vi "SetIncrementTime.vi"(8 "error in":errorcluster, 11 "Cycles":T1={"DELICATE"=10.0, "LOW"=10.0, "MEDIUM"=10.0, "HIGH"=10.0} {"HIGH" min=0.0 max=90.0 step=1.0; "MEDIUM" min=0.0 max=90.0 step=1.0; "LOW" min=0.0 max=90.0 step=1.0; "DELICATE" min=0.0 max=90.0 step=1.0}) -> (0 "error out":errorcluster, 3 "TimeData":string)   [LabVIEW 2023]
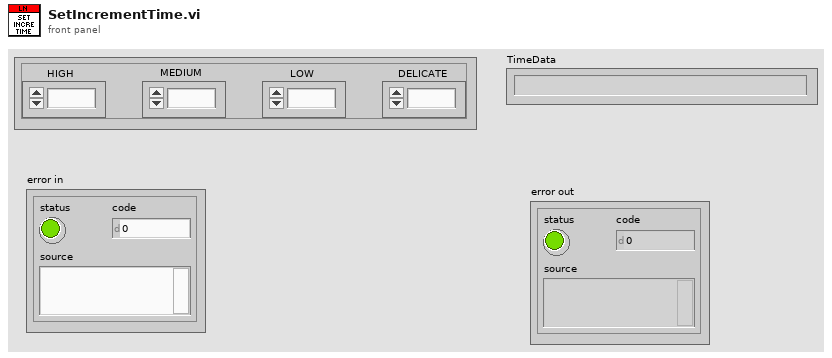
[diagram p1: front panel]
types:
  T1 = cluster{"DELICATE":dbl, "LOW":dbl, "MEDIUM":dbl, "HIGH":dbl}
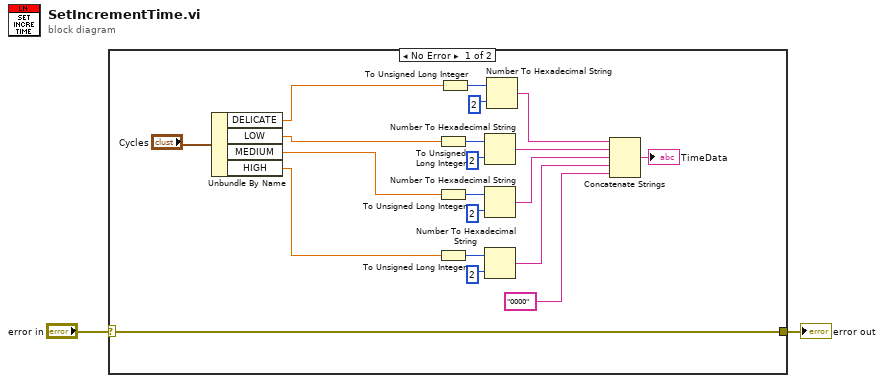
[diagram p0: block diagram]
diagram:
  n1 = case shown="No Error" "error in" {
    selector: "error in" -> [w3 w23]
    tunnel: [w3 w23] -> w1
    frame No Error {
      n2 = Unbundle By Name("Cycles") -> ("DELICATE"=w7:dbl, "LOW"=w6:dbl, "MEDIUM"=w5:dbl, "HIGH"=w4:dbl)
      n3 = To Unsigned Long Integer(number=w6) -> (unsigned 32bit integer=w20:u32)
      n4 = To Unsigned Long Integer(number=w5) -> (unsigned 32bit integer=w17:u32)
      n5 = To Unsigned Long Integer(number=w4) -> (unsigned 32bit integer=w16:u32)
      n6 = To Unsigned Long Integer(number=w7) -> (unsigned 32bit integer=w21:u32)
      n7 = Number To Hexadecimal String(1:i16 2 ("width (-)"), 2:w20) -> (0:w13:string)
      n8 = Number To Hexadecimal String(1:i16 2 ("width (-)"), 2:w17) -> (0:w12:string)
      n9 = Number To Hexadecimal String(1:i16 2 ("width (-)"), 2:w16) -> (0:w11:string)
      n10 = Number To Hexadecimal String(1:i16 2 ("width (-)"), 2:w21) -> (0:w14:string)
      n11 = Concatenate Strings(w14, w13, w12, w11, "0000" ("string")) -> (→"TimeData":string)
    }
    frame Error {
    }
  }
  "error out" <- w1
